vi "Initialize (Remote No Resource).vi"(1 "https?":bool, 5 "Hostname/IP":string, 7 "Port":u16, 11 "error in (no error)":errorcluster, 12 "username":string="admin", 13 "password":string) -> (4 "SLSC Remote out":refnum<class "SLSC Remote.lvclass">, 15 "error out":errorcluster)   [LabVIEW 2015, in "SLSC Remote.lvclass"]
uses:
  SLSC Remote.lvclass
  SLSC Interface Class/slsc type.ctl
  <vilib>/SLSC/Initialize Session without Resources.vi
  SLSC Interface Class/SLSC Interface.lvclass
  <vilib>/SLSC/SLSC.lvlib
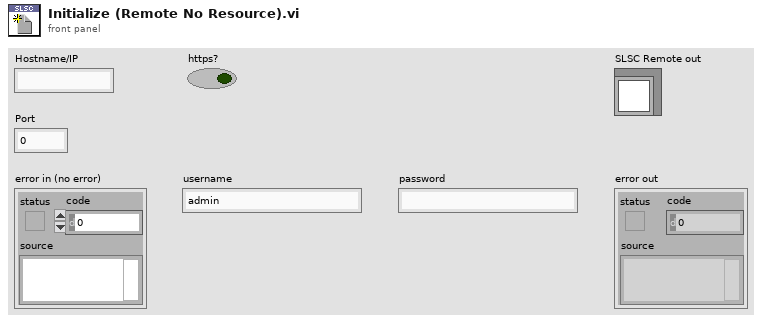
[diagram p1: front panel]
types:
  T1 = typedef "SLSC Interface.lvclass/slsc type.ctl" = enum16{"device", "nvmem", "channel", "none"}
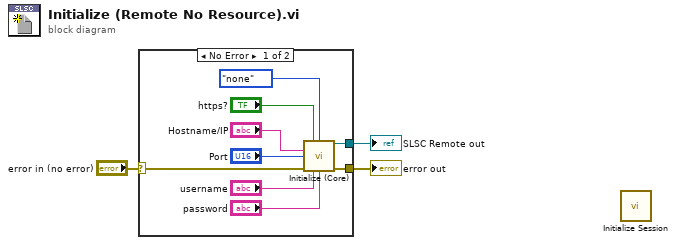
[diagram p0: block diagram]
diagram:
  n1 = case shown="No Error" "error in (no error)" {
    selector: "error in (no error)" -> [w8 w13]
    tunnel: [w6 w13] -> w2
    tunnel: [w7 _] -> w1
    frame No Error {
      n2 = call "Initialize (Core).vi"("https?"="https?", "slsc type"=slsc_type."none", "Hostname/IP"="Hostname/IP", "Port"="Port", "error in (no error)"=w8, "username"="username", "password"="password") -> ("SLSC Remote out"=w7:refnum<class "SLSC Remote.lvclass">, "error out"=w6:errorcluster)  [unwired: 7 in]
    }
    frame Error {
    }
  }
  "error out" <- w2
  "SLSC Remote out" <- w1
  n3 = call-poly <vilib>:"Initialize Session.vi"() -> ()  [unwired: 14 in, 2 out]
